vi "Set Dialog Types.vi"(0 "Test Executive Builder in":refnum<class "Test Executive Builder.lvclass">, 7 "Subroutine Dialog Type":refnum<class "ITest Executive Builder Dialog.lvclass">, 9 "Test Step Dialog Type":refnum<class "ITest Executive Builder Dialog.lvclass">, 11 "Name Only Dialog Type":refnum<class "ITest Executive Builder Dialog.lvclass">, 12 "Sequence Dialog Type":refnum<class "ITest Executive Builder Dialog.lvclass">, 13 "Conditional Dialog Type":refnum<class "ITest Executive Builder Dialog.lvclass">, 14 "For Loop Dialog Type":refnum<class "ITest Executive Builder Dialog.lvclass">) -> (4 "Test Executive Builder out":refnum<class "Test Executive Builder.lvclass">)   [LabVIEW 2017, in "Test Executive Builder.lvclass"]
uses:
  <vilib>/gpm_packages/@cs/Test-executive-builder/Example/Application/Test Executive Builder/Test Executive Builder/Test Executive Builder.lvclass
  <vilib>/gpm_packages/@cs/Test-executive-builder/Source/Test Executive Builder Dialogs/ITest Executive Builder Dialog/ITest Executive Builder Dialog.lvclass
  <vilib>/gpm_packages/@cs/Test-executive-builder/Example/Application/Test Executive Builder/Test Executive Builder/Test Executive Builder.lvclass/Test Executive Builder.ctl
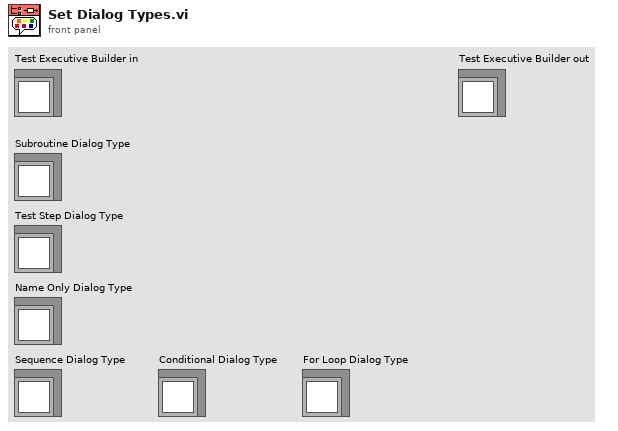
[diagram p1: front panel]
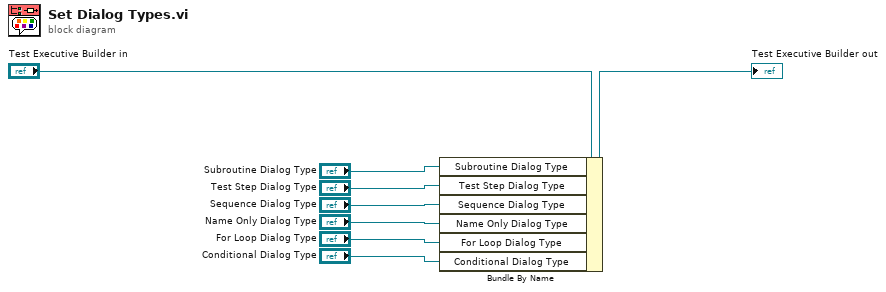
[diagram p0: block diagram]
diagram:
  n1 = Bundle By Name(cluster="Test Executive Builder in", "Subroutine Dialog Type"="Subroutine Dialog Type", "Test Step Dialog Type"="Test Step Dialog Type", "Sequence Dialog Type"="Sequence Dialog Type", "Name Only Dialog Type"="Name Only Dialog Type", "For Loop Dialog Type"="For Loop Dialog Type", "Conditional Dialog Type"="Conditional Dialog Type") -> (→"Test Executive Builder out":refnum<class "Test Executive Builder.lvclass">)
